vi "NI-DCPower Pulse Voltage Sequence.vi"() -> ()   [LabVIEW 2021]
doc: "Demonstrates how to use the DCPower Pulse API to generate a Voltage Pulse Sequence. This example initializes a session, configures the Source Mode and the Output Function, configures the pulse parameters, initiates the pulse output sequence, and takes measurements."
uses:
  <instrlib>/niDCPower/nidcpower.llb/niDCPower Output Function.ctl
  <instrlib>/niDCPower/nidcpower.llb/niDCPower Source Mode.ctl
  <instrlib>/niDCPower/nidcpower.llb/niDCPower Aperture Time Units.ctl
  <instrlib>/niDCPower/nidcpower.llb/niDCPower Wait For Event - Event.ctl
panel:
  in  "Pulse Current Limit Range":dbl=0.1 format="%#.6p"
  in  "Pulse Bias Voltage Level":dbl format="%.5p"
  in  "Pulse Voltage Level Range":dbl=6.0 format="%#.6p"
  in  "Pulse Current Limit":dbl=0.1 format="%.5p"
  in  "Pulse Bias Current Limit":dbl=0.1 format="%.5p"
  in  "Pulse Voltage Sequence":dbl[](array[numeric])=[1.0, 2.0, 3.0] format="%_6g"
  in  "Source Delays":dbl[](array[numeric])=[5e-05, 6e-05, 7e-05] format="%.3p"
  in  "Aperture Time (Sec)":dbl=0.0001
  out "Current Measurements":dbl[](array[numeric])
  out "Voltage Measurements":dbl[](array[numeric])
  in  "Pulse Bias Delay (Sec)":dbl=1e-06 format="%.3p"
  in  "Pulse Off Time (Sec)":dbl=0.005
  in  "Pulse On Time (Sec)":dbl=0.001
  in  "Load SMUs":refnum<k15>="Dev1" caption="Load SMU"
  in  "Load SMU Channel":string="0"
  # "Overview: This example outputs a sequence of voltage pulses and takes a voltage and current measurement at the peak of each pulse. \nRequirements: NI-DCPower\nInstructions:\n1. Select the appropriate device in the Resource Name control.\n2. Configure the pulse sequence that you would like to output.\n3. Run the VI."
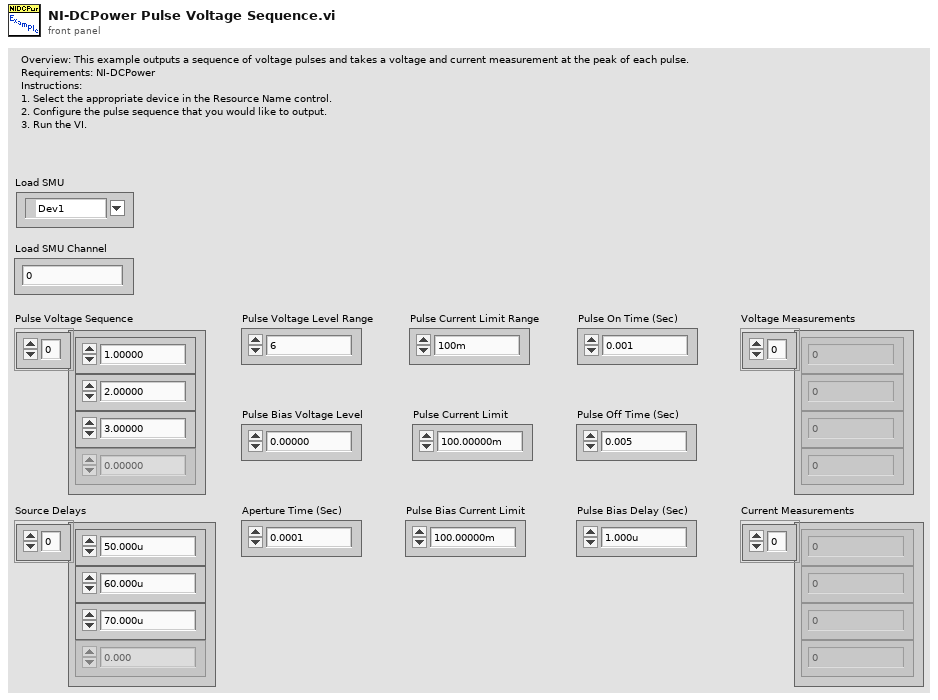
[diagram p1: front panel]
types:
  T1 = typedef "niDCPower Wait For Event - Event.ctl" = i32
  T2 = typedef "niDCPower Output Function.ctl" = i32
  T3 = typedef "niDCPower Aperture Time Units.ctl" = i32
  T4 = typedef "niDCPower Source Mode.ctl" = i32
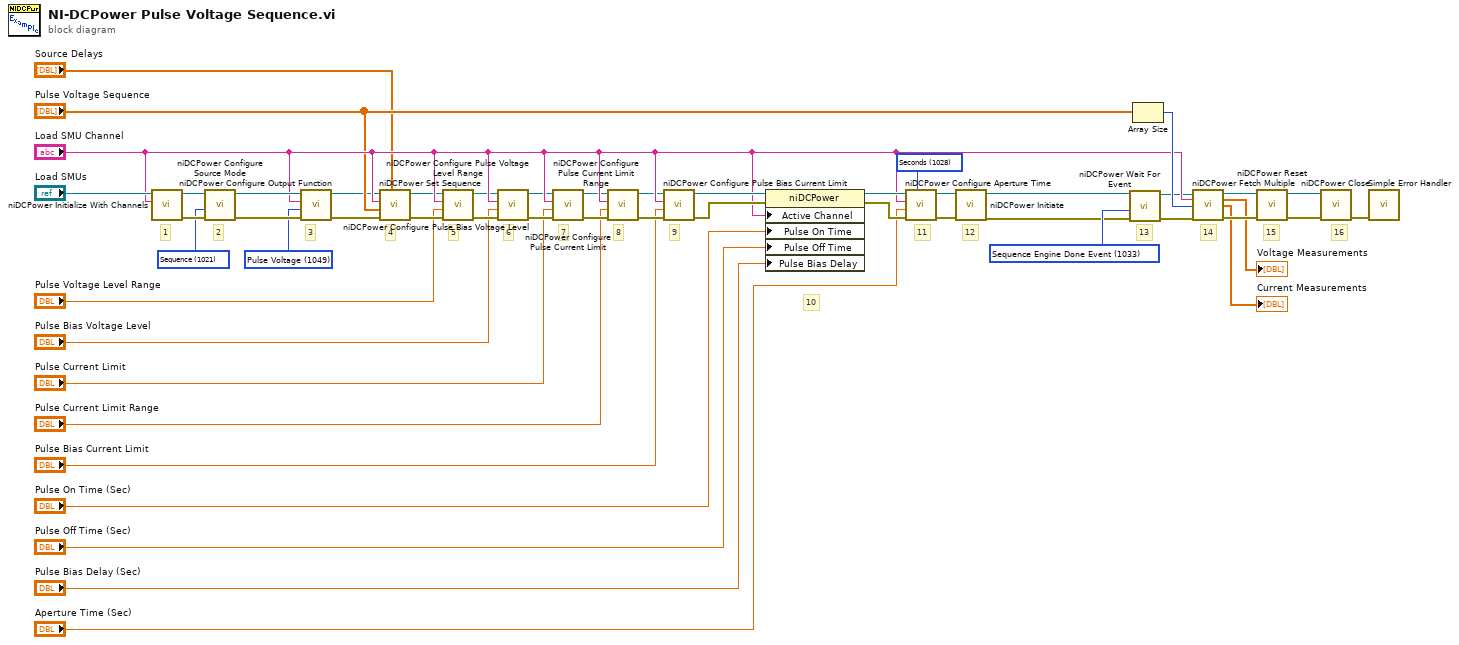
[diagram p0: block diagram]
diagram:
  w5 = T1 1033 items=["Source Complete Event"=1030, "Measure Complete Event"=1031, "Sequence Iteration Complete Event"=1032, "Sequence Engine Done Event"=1033, "Pulse Complete Event"=1051, "Ready For Pulse Trigger Event"=1052] ("event")
  w15 = T2 1049 items=["DC Voltage"=1006, "DC Current"=1007, "Pulse Voltage"=1049, "Pulse Current"=1050] ("output function")
  w28 = T3 1028 items=["Seconds"=1028, "Powerline Cycles"=1029] ("aperture time units")
  w47 = T4 1021 items=["Single Point"=1020, "Sequence"=1021] ("source mode")
  # "15"
  # "9"
  # "8"
  # "7"
  # "6"
  # "5"
  # "4"
  # "3"
  # "16"
  # "14"
  # "13"
  # "12"
  # "11"
  # "10"
  # "2"
  # "1"
  n1 = call <instrlib>:"niDCPower Initialize With Channels.vi"("channels"="Load SMU Channel", "resource name"="Load SMUs") -> ("error out"=w51:errorcluster, "instrument handle out"=w44:refnum<k15>)  [unwired: 3 in, 5 out]
  n2 = call <instrlib>:"niDCPower Configure Source Mode.vi"("error in (no error)"=w51, "source mode"=w47, "instrument handle"=w44) -> ("error out"=w45:errorcluster, "instrument handle out"=w46:refnum<k15>)  [unwired: 7 out]
  n3 = call <instrlib>:"niDCPower Configure Output Function.vi"("error in (no error)"=w45, "output function"=w15, "channel name"="Load SMU Channel", "instrument handle"=w46) -> ("error out"=w7:errorcluster, "instrument handle out"=w9:refnum<k15>)  [unwired: 6 out]
  n4 = call <instrlib>:"niDCPower Set Sequence.vi"("source delays"="Source Delays", "error in (no error)"=w7, "values"="Pulse Voltage Sequence", "channel name"="Load SMU Channel", "instrument handle"=w9) -> ("error out"=w24:errorcluster, "instrument handle out"=w8:refnum<k15>)  [unwired: 5 in]
  n5 = call <instrlib>:"niDCPower Configure Pulse Voltage Level Range.vi"("error in (no error)"=w24, "pulse voltage level range"="Pulse Voltage Level Range", "channel name"="Load SMU Channel", "instrument handle"=w8) -> ("error out"=w23:errorcluster, "instrument handle out"=w22:refnum<k15>)  [unwired: 6 in]
  n6 = call <instrlib>:"niDCPower Configure Pulse Bias Voltage Level.vi"("error in (no error)"=w23, "pulse bias voltage level"="Pulse Bias Voltage Level", "channel name"="Load SMU Channel", "instrument handle"=w22) -> ("error out"=w21:errorcluster, "instrument handle out"=w20:refnum<k15>)  [unwired: 6 in]
  n7 = call <instrlib>:"niDCPower Configure Pulse Current Limit.vi"("error in (no error)"=w21, "pulse current limit"="Pulse Current Limit", "channel name"="Load SMU Channel", "instrument handle"=w20) -> ("error out"=w19:errorcluster, "instrument handle out"=w18:refnum<k15>)  [unwired: 6 in]
  n8 = call <instrlib>:"niDCPower Configure Pulse Current Limit Range.vi"("error in (no error)"=w19, "pulse current limit range"="Pulse Current Limit Range", "channel name"="Load SMU Channel", "instrument handle"=w18) -> ("error out"=w17:errorcluster, "instrument handle out"=w16:refnum<k15>)  [unwired: 6 in]
  n9 = call <instrlib>:"niDCPower Configure Pulse Bias Current Limit.vi"("error in (no error)"=w17, "pulse bias current limit"="Pulse Bias Current Limit", "channel name"="Load SMU Channel", "instrument handle"=w16) -> ("error out"=w38:errorcluster, "instrument handle out"=w39:refnum<k15>)  [unwired: 6 in]
  n10 = property class="niDCPower"(reference=w39, error in=w38, "Active Channel"="Load SMU Channel", "Pulse On Time"="Pulse On Time (Sec)", "Pulse Off Time"="Pulse Off Time (Sec)", "Pulse Bias Delay"="Pulse Bias Delay (Sec)") -> (reference out=w30:refnum<k15>, error out=w32:errorcluster)
  n11 = call <instrlib>:"niDCPower Configure Aperture Time.vi"("aperture time units"=w28, "error in (no error)"=w32, "aperture time"="Aperture Time (Sec)", "channel name"="Load SMU Channel", "instrument handle"=w30) -> ("error out"=w31:errorcluster, "instrument handle out"=w29:refnum<k15>)  [unwired: 5 in]
  n12 = call <instrlib>:"niDCPower Initiate.vi"("error in (no error)"=w31, "instrument handle"=w29) -> ("error out"=w1:errorcluster, "instrument handle out"=w2:refnum<k15>)  [unwired: 2 in, 6 out]
  n13 = call <instrlib>:"niDCPower Wait For Event.vi"("error in (no error)"=w1, "event"=w5, "instrument handle"=w2) -> ("error out"=w3:errorcluster, "instrument handle out"=w4:refnum<k15>)  [unwired: 7 in]
  n14 = Array Size(array="Pulse Voltage Sequence") -> (size(s)=w33:i32)
  n15 = call <instrlib>:"niDCPower Fetch Multiple.vi"("instrument handle"=w4, "channel name"="Load SMU Channel", "count (1)"=w33, "error in (no error)"=w3) -> ("instrument handle out"=w35:refnum<k15>, "voltage measurements"=→"Voltage Measurements":dbl[], "current measurements"=→"Current Measurements":dbl[], "error out"=w50:errorcluster)  [unwired: 6 in, 2 out]
  n16 = call <instrlib>:"niDCPower Reset.vi"("error in (no error)"=w50, "instrument handle"=w35) -> ("error out"=w42:errorcluster, "instrument handle out"=w41:refnum<k15>)  [unwired: 2 in, 6 out]
  n17 = call <instrlib>:"niDCPower Close.vi"("error in (no error)"=w42, "instrument handle"=w41) -> ("error out"=w43:errorcluster)  [unwired: 9 out]
  n18 = call <vilib>:"Simple Error Handler.vi"("error in (no error)"=w43) -> ()  [unwired: 1 in, 8 out]
